vi "PopulateChannelArray.vi"(1 "Update size?":bool=TRUE, 2 "error in":errorcluster, 3 "Channel Selection ref":refnum<vi>, 4 "Enum in":refnum<vi>) -> (0 "error out":errorcluster)   [LabVIEW 2015]
doc: "Populates the channel selection array with options for channels"
uses:
  controls/ChannelSelection.ctl
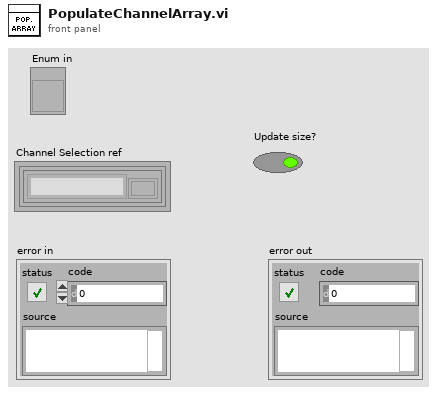
[diagram p1: front panel]
types:
  T1 = typedef "ChannelSelection.ctl" = cluster{"Channel name":string, "Enum id":u16, "Logging?":bool}[]
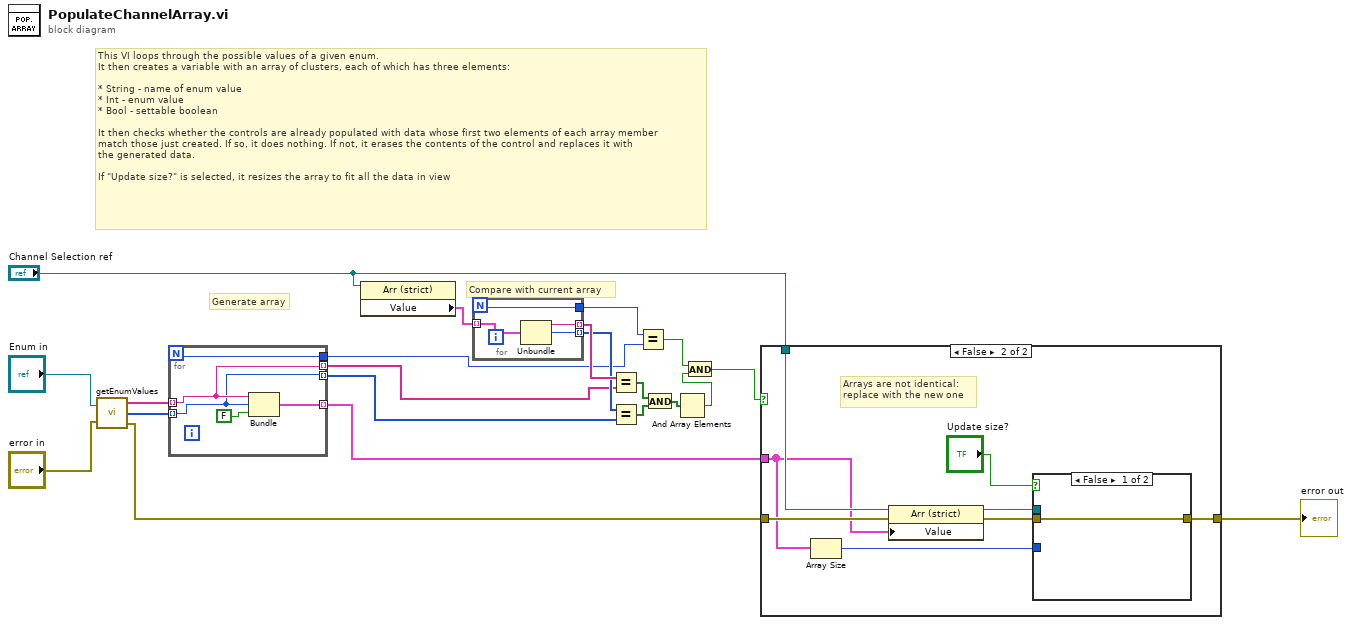
[diagram p0: block diagram]
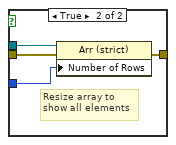
[diagram p3: hidden frame]
diagram:
  # "Compare with current array"
  # "Generate array"
  # "This VI loops through the possible values of a given enum.\nIt then creates a variable with an array of clusters, each of which has three elements:\n\n* String - name of enum value\n* Int - enum value\n* Bool - settable boolean\n\nIt then checks whether the controls are already populated with data whose first two elements of each array member\nmatch those just created. If so, it does nothing. If not, it erases the contents of the control and replaces it with \nthe generated data.\n\nIf \"Update size?\" is selected, it resizes the array to fit all the data in view"
  n1 = call "getEnumValues.vi"("Enum reference"="Enum in", "error in (no error)"="error in") -> ("Enum labels"=w18:string[], "Enum values"=w17:u16[], "error out"=w21:errorcluster)
  n2 = for {
    N -> [w22]
    tunnel: w18 -> [w24] mode=indexing
    tunnel: w17 -> [w23] mode=indexing
    tunnel: [w25] -> w6 mode=indexing
    tunnel: [w24] -> w7 mode=indexing
    tunnel: [w23] -> w12 mode=indexing
    tunnel: [w22] -> w4
    n3 = Bundle(w24, w23, FALSE) -> (w25:cluster{string, u16, bool})  [unwired: 1 in]
  }
  n4 = property class="Arr (strict)"(reference="Channel Selection ref") -> ("Value"=w15:T1)  [unwired: 1 in, 2 out]
  n5 = for {
    N -> [w27]
    tunnel: w15 -> [w30] mode=indexing
    tunnel: [w29] -> w14 mode=indexing
    tunnel: [w28] -> w13 mode=indexing
    tunnel: [w27] -> w5
    n6 = Unbundle(w30) -> ("Channel name"=w29:string, "Enum id"=w28:u16)  [unwired: 1 out]
  }
  n7 = Equal?(x=w14, y=w7) -> (x = y?=w11:bool[])
  n8 = Equal?(x=w13, y=w12) -> (x = y?=w10:bool[])
  n9 = Equal?(x=w5, y=w4) -> (x = y?=w2:bool)
  n10 = And(x=w11, y=w10) -> (x .and. y?=w9:bool[])
  n11 = And Array Elements(Boolean array=w9) -> (logical AND=w3:bool)
  n12 = And(x=w2, y=w3) -> (x .and. y?=w1:bool)
  n13 = case shown="False" w1 {
    tunnel: w21 -> [w31 w39]
    tunnel: "Channel Selection ref" -> [_ w38]
    tunnel: [w31 w33] -> w8
    tunnel: w6 -> [_ w37]
    frame True {
      # "Arrays are identical: don't update anything"
      # "Resize array to show all elements"
    }
    frame False {
      # "Arrays are not identical:\nreplace with the new one"
      n14 = Array Size(array=w37) -> (size(s)=w34:i32)
      n15 = property on="Property Node" class="Arr (strict)"(reference=w38, error in=w39, "Value"=w37) -> (reference out=w35:refnum<vi>, error out=w36:errorcluster)
      n16 = case shown="False" "Update size?" {
        tunnel: w36 -> [w40 w44]
        tunnel: w35 -> [_ w43]
        tunnel: w34 -> [_ w42]
        tunnel: [w40 w41] -> w33
        frame False {
        }
        frame True {
          # "Resize array to\nshow all elements"
          n17 = property on="Property Node" class="Arr (strict)"(reference=w43, error in=w44, "Number of Rows"=w42) -> (error out=w41:errorcluster)  [unwired: 1 out]
        }
      }
    }
  }
  "error out" <- w8
